vi "PH_O2_Watch.ProcCases.vi"(0 "i ref in":refnum<vi>, 1 "selector":string, 2 "Data":T1, 3 "call cluster":T2={"Object"="", "Selector"="", "CallType"=enum."synchronous", "Async Object"="", "Async Selector"="", "Data Descriptor"="", "Data"=[], "Error #"=0, "Expire"=0}, 5 "error in (no error)":errorcluster) -> (14 "i ref out":refnum<vi>, 17 "answer cluster":T2={"Object"="", "Selector"="", "CallType"=enum."synchronous", "Async Object"="", "Async Selector"="", "Data Descriptor"="", "Data"=[], "Error #"=0, "Expire"=0}, 19 "error out":errorcluster)   [LabVIEW 2014, in "PH_O2_Watch.lvlib"]
doc: "This method is called by a process from within the default case in the event loop. The methods of a class that are linked to events will be called from THIS method. Add your code here."
uses:
  PH_O2_Watch.lvlib
  CSCore/CSSystem/CoreDefs/CoreDefs.call_type.ctl
  CSCore/BaseProcess/BaseProcess.descriptor string definition.ctl
  CSCore/CSSystem/CoreDefs/CoreDefs.rawDataType.ctl
  CSCore/CSSystem/CoreLib/CoreLib.string 2 byte array.vi
  CSCore/CSSystem/CoreLib/CoreLib.byte array 2 double.vi
  CSCore/BaseProcess/BaseProcess.lvlib
  PH_Common/PH_Common.lvlib
  CSCore/CSSystem/CoreLib/CoreLib.lvlib
  CSCore/CAEObj/CAEObj.lvlib
  PH_PSDBWriter/PH_PSDBWriter.lvlib
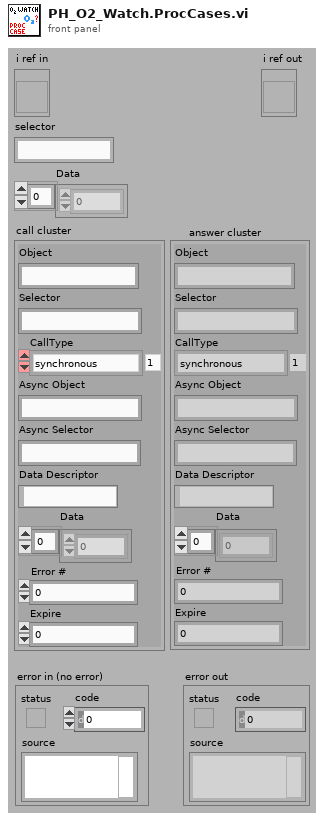
[diagram p1: front panel]
types:
  T1 = typedef "CoreDefs.rawDataType.ctl" = i8[]
  T2 = typedef "CoreDefs.call_type.ctl" = cluster{"Object":string, "Selector":string, "CallType":enum16{"simple", "synchronous", "asynchronous"}, "Async Object":string, "Async Selector":string, "Data Descriptor":T3, "Data":T1, "Error #":i32, "Expire":u32}
  T3 = typedef "BaseProcess.lvlib/BaseProcess.descriptor string definition.ctl" = string
  T4 = typedef "PH_StatusHandler.lvlib/PH_StatusHandler.Status.ctl" = i16
  T5 = typedef "PH_O2_Watch.lvlib/PH_O2_Watch.i attribute.ctl" = cluster{"GUI Refs":cluster{"PreAlert":refnum<vi>, "Alert":refnum<vi>, "Failure":refnum<vi>, "Concentration":refnum<vi>, "Delete":refnum<vi>, "Limit":refnum<vi>}, "State PreAlert":T4, "State Alert":T4, "State Failure":T4, "Concentration":dbl, "Limit":dbl}
  T6 = typedef "PH_PSDBWriter.lvlib/PH_PSDBWriter.PHELIX-Subsystems.ctl" = i32
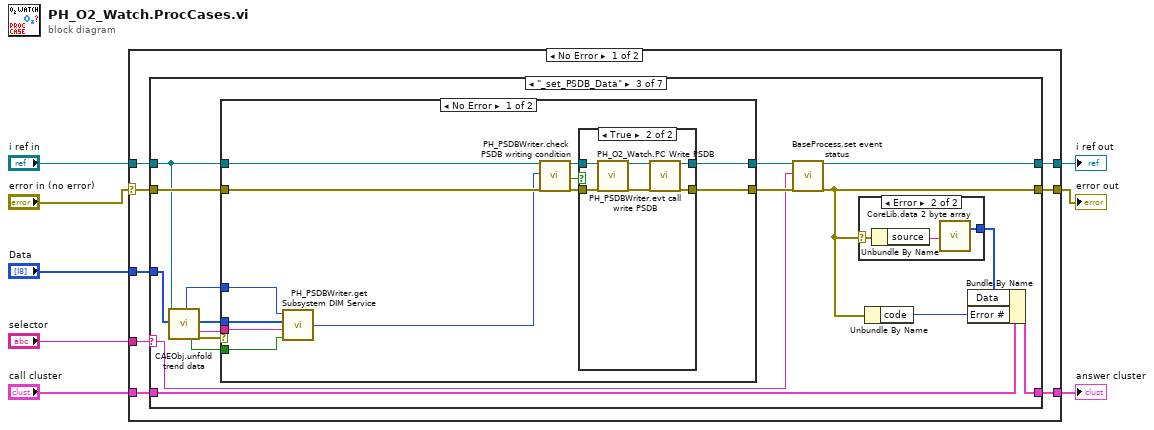
[diagram p0: block diagram]
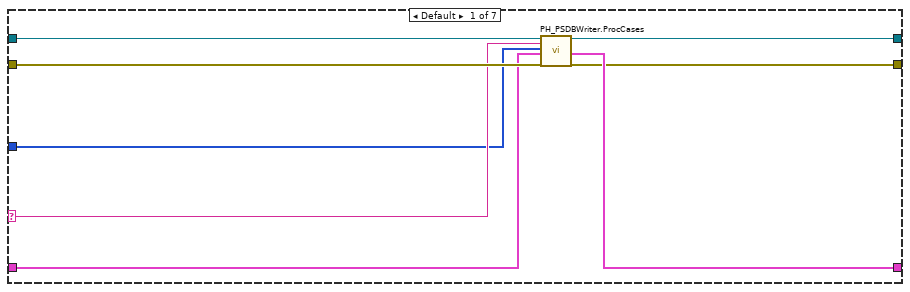
[diagram p2: hidden frame]
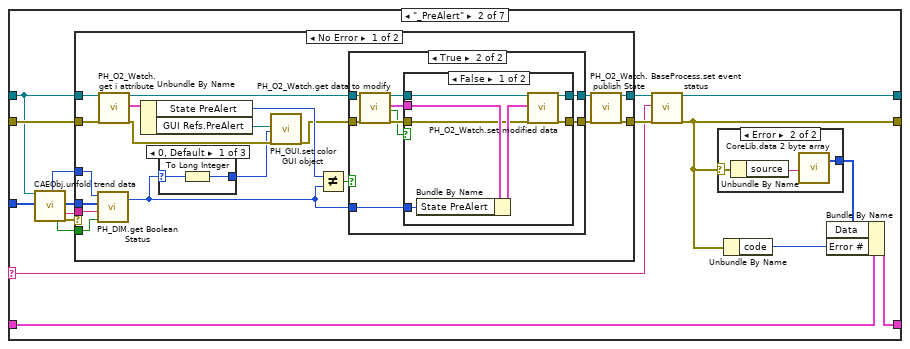
[diagram p3: hidden frame]
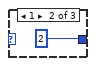
[diagram p5: hidden frame]
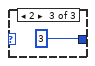
[diagram p6: hidden frame]
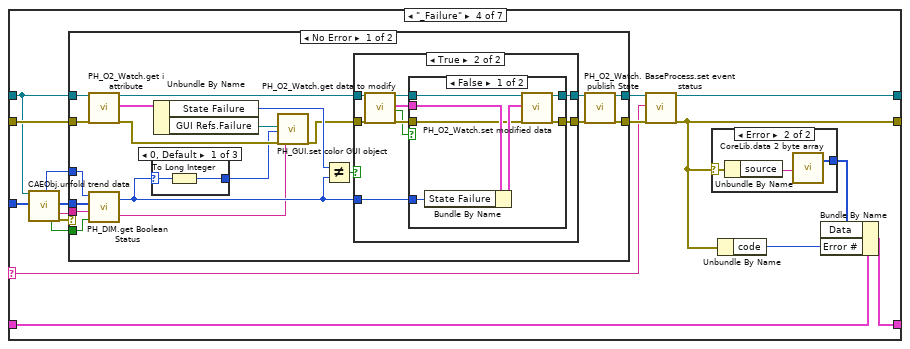
[diagram p13: hidden frame]
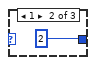
[diagram p15: hidden frame]
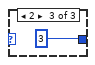
[diagram p16: hidden frame]
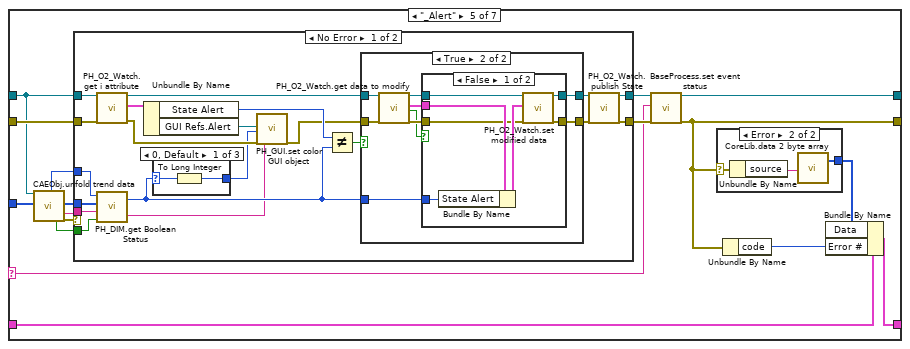
[diagram p20: hidden frame]
diagram:
  n1 = case shown="No Error" "error in (no error)" {
    selector: "error in (no error)" -> [w9 w384]
    tunnel: "selector" -> [w16 _]
    tunnel: [w15 w383] -> w7
    tunnel: "call cluster" -> [w14 w383]
    tunnel: "i ref in" -> [w13 w385]
    tunnel: "Data" -> [w12 _]
    tunnel: [w11 w385] -> w3
    tunnel: [w10 w384] -> w2
    frame No Error {
      n2 = case shown="\"_set_PSDB_Data\"" w16 {
        selector: w16 -> [w21 w30 w90 w138 w203 w268 w332]
        tunnel: w13 -> [w20 w31 w96 w137 w204 w270 w336]
        tunnel: w14 -> [w22 w28 w94 w135 w201 w266 w331]
        tunnel: [w23 w29 w95 w136 w202 w267 w335] -> w15
        tunnel: w9 -> [w24 w32 w97 w139 w205 w271 w337]
        tunnel: w12 -> [w19 w27 w93 w134 w200 w269 _]
        tunnel: [w18 w26 w92 w133 w199 w265 w334] -> w11
        tunnel: [w17 w25 w91 w132 w198 w264 w333] -> w10
        frame Default {
          n3 = call "PH_PSDBWriter.ProcCases.vi"("i ref in"=w20, "selector"=w21, "Data"=w19, "call cluster"=w22, "error in"=w24) -> ("i ref out"=w18:refnum<vi>, "answer cluster"=w23:T2, "error out"=w17:errorcluster)  [unwired: 12 in]
        }
        frame "_PreAlert" {
          n4 = call "CAEObj.unfold trend data.vi"("i ref in"=w31, "raw trend data"=w27) -> ("quality"=w38:i32, "no link"=w37:bool, "data"=w39:i8[], "typeDescriptor"=w40:string, "error out"=w41:errorcluster)  [unwired: 9 in, 4 out]
          n5 = case shown="No Error" w41 {
            tunnel: [w52 w89] -> w34
            tunnel: w31 -> [w58 w89]
            tunnel: w32 -> [w63 w88]
            tunnel: [w50 w88] -> w33
            tunnel: w40 -> [w62 _]
            tunnel: w39 -> [w61 _]
            tunnel: w38 -> [w60 _]
            tunnel: w37 -> [w59 _]
            frame No Error {
              n6 = call "PH_DIM.get Boolean Status.vi"("no link"=w59, "typeDescriptor"=w62, "data"=w61, "quality"=w60) -> ("Status"=w46:T4)  [unwired: 1 out]
              n7 = call "PH_O2_Watch.get i attribute.vi"("i ref in"=w58, "error in (no error)"=w63) -> ("i ref out"=w57:refnum<vi>, "i attribute"=w56:T5, "error out"=w48:errorcluster)  [unwired: 15 in]
              n8 = Unbundle By Name(w56) -> ("State PreAlert"=w55:T4, "GUI Refs.PreAlert"=w49:refnum<vi>)
              n9 = case shown="0, Default" w46 {
                selector: w46 -> [w65 _ _]
                tunnel: [w64 2 3] -> w45
                frame 0, Default {
                  n10 = To Long Integer(number=w65) -> (32bit integer=w64:i32)
                }
                frame 1 {
                }
                frame 2 {
                }
              }
              n11 = call "PH_GUI.set color GUI object.vi"("GUI object Ref"=w49, "State"=w45, "error in (no error)"=w48) -> ("error out"=w47:errorcluster)  [unwired: 16 in]
              n12 = Not Equal?(x=w55, y=w46) -> (x != y?=w54:bool)
              n13 = case shown="True" w54 {
                tunnel: w46 -> [_ w74]
                tunnel: [w69 w71] -> w51
                tunnel: [w68 w70] -> w53
                tunnel: w47 -> [w68 w73]
                tunnel: w57 -> [w69 w72]
                frame False {
                }
                frame True {
                  n14 = call "PH_O2_Watch.get data to modify.vi"("i ref in"=w72, "error in (no error)"=w73) -> ("i ref out"=w77:refnum<vi>, "i attribute"=w78:T5, "timed out"=w75:bool, "error out"=w76:errorcluster)  [unwired: 14 in]
                  n15 = case shown="False" w75 {
                    tunnel: w78 -> [w82 _]
                    tunnel: w74 -> [w80 _]
                    tunnel: [w85 w86] -> w70
                    tunnel: w77 -> [w84 w87]
                    tunnel: [w83 w87] -> w71
                    tunnel: w76 -> [w79 w86]
                    frame False {
                      n16 = Bundle By Name(cluster=w82, "State PreAlert"=w80) -> (w81:T5)
                      n17 = call "PH_O2_Watch.set modified data.vi"("i ref in"=w84, "i attribute"=w81, "error in (no error)"=w79) -> ("i ref out"=w83:refnum<vi>, "error out"=w85:errorcluster)  [unwired: 15 in]
                    }
                    frame True {
                    }
                  }
                }
              }
              n18 = call "PH_O2_Watch.publish State.vi"("i ref in"=w51, "error in (no error)"=w53) -> ("i ref out"=w52:refnum<vi>, "error out"=w50:errorcluster)  [unwired: 16 in]
            }
            frame Error {
            }
          }
          n19 = call "BaseProcess.set event status.vi"("i ref in"=w34, "EventStatus"=w30, "error in (no error)"=w33) -> ("i ref out"=w26:refnum<vi>, "error out"=w25:errorcluster)  [unwired: 14 in, 1 out]
          n20 = case shown="Error" w25 {
            selector: w25 -> [_ w44]
            tunnel: [_ w42] -> w35
            frame No Error {
            }
            frame Error {
              n21 = Unbundle By Name(w44) -> ("source"=w43:string)
              n22 = call-poly "CoreLib.data 2 byte array.vi"("string"=w43) -> ("byteArray out"=w42:T1)  [unwired: 18 in]
            }
          }
          n23 = Unbundle By Name(w25) -> ("code"=w36:i32)
          n24 = Bundle By Name(cluster=w28, "Data"=w35, "Error #"=w36) -> (w29:T2)
        }
        frame "_set_PSDB_Data" {
          n25 = call "CAEObj.unfold trend data.vi"("i ref in"=w96, "raw trend data"=w93) -> ("quality"=w103:i32, "no link"=w102:bool, "data"=w104:i8[], "typeDescriptor"=w105:string, "error out"=w106:errorcluster)  [unwired: 9 in, 4 out]
          n26 = case shown="No Error" w106 {
            tunnel: [w121 w131] -> w99
            tunnel: w96 -> [w117 w131]
            tunnel: w97 -> [w119 w130]
            tunnel: [w120 w130] -> w98
            tunnel: w105 -> [w113 _]
            tunnel: w104 -> [w114 _]
            tunnel: w103 -> [w111 _]
            tunnel: w102 -> [w112 _]
            frame No Error {
              n27 = call "PH_PSDBWriter.get Subsystem DIM Service.vi"("no link"=w112, "typeDescriptor"=w113, "data"=w114, "quality"=w111) -> ("PHELIX Subsystems"=w110:T6)
              n28 = call "PH_PSDBWriter.check PSDB writing condition.vi"("i ref in"=w117, "wanted Subsystem"=w110, "error IO"=w119) -> ("i ref out"=w116:refnum<vi>, "write PSDB?"=w115:bool, "error out"=w118:errorcluster)  [unwired: 14 in]
              n29 = case shown="True" w115 {
                tunnel: [w123 w129] -> w121
                tunnel: [w122 w128] -> w120
                tunnel: w116 -> [w123 w127]
                tunnel: w118 -> [w122 w125]
                frame False {
                }
                frame True {
                  n30 = call "PH_O2_Watch.PC Write PSDB.vi"("i ref in"=w127, "error IO"=w125) -> ("i ref out"=w126:refnum<vi>, "error out"=w124:errorcluster)  [unwired: 16 in]
                  n31 = call "PH_PSDBWriter.evt call write PSDB.vi"("i ref in"=w126, "error in (no error)"=w124) -> ("i ref out"=w129:refnum<vi>, "error out"=w128:errorcluster)  [unwired: 16 in]
                }
              }
            }
            frame Error {
            }
          }
          n32 = call "BaseProcess.set event status.vi"("i ref in"=w99, "EventStatus"=w90, "error in (no error)"=w98) -> ("i ref out"=w92:refnum<vi>, "error out"=w91:errorcluster)  [unwired: 14 in, 1 out]
          n33 = case shown="Error" w91 {
            selector: w91 -> [_ w109]
            tunnel: [_ w107] -> w100
            frame No Error {
            }
            frame Error {
              n34 = Unbundle By Name(w109) -> ("source"=w108:string)
              n35 = call-poly "CoreLib.data 2 byte array.vi"("string"=w108) -> ("byteArray out"=w107:T1)  [unwired: 18 in]
            }
          }
          n36 = Unbundle By Name(w91) -> ("code"=w101:i32)
          n37 = Bundle By Name(cluster=w94, "Data"=w100, "Error #"=w101) -> (w95:T2)
        }
        frame "_Failure" {
          n38 = call "CAEObj.unfold trend data.vi"("i ref in"=w137, "raw trend data"=w134) -> ("quality"=w145:i32, "no link"=w144:bool, "data"=w146:i8[], "typeDescriptor"=w147:string, "error out"=w148:errorcluster)  [unwired: 9 in, 4 out]
          n39 = case shown="No Error" w148 {
            tunnel: [w161 w197] -> w141
            tunnel: w137 -> [w166 w197]
            tunnel: w139 -> [w171 w196]
            tunnel: [w159 w196] -> w140
            tunnel: w147 -> [w170 _]
            tunnel: w146 -> [w169 _]
            tunnel: w145 -> [w168 _]
            tunnel: w144 -> [w167 _]
            frame No Error {
              n40 = call "PH_O2_Watch.get i attribute.vi"("i ref in"=w166, "error in (no error)"=w171) -> ("i ref out"=w165:refnum<vi>, "i attribute"=w164:T5, "error out"=w156:errorcluster)  [unwired: 15 in]
              n41 = call "PH_DIM.get Boolean Status.vi"("no link"=w167, "typeDescriptor"=w170, "data"=w169, "quality"=w168) -> ("further information"=w152:string, "Status"=w154:T4)
              n42 = case shown="0, Default" w154 {
                selector: w154 -> [w173 _ _]
                tunnel: [w172 2 3] -> w153
                frame 0, Default {
                  n43 = To Long Integer(number=w173) -> (32bit integer=w172:i32)
                }
                frame 1 {
                }
                frame 2 {
                }
              }
              n44 = Unbundle By Name(w164) -> ("State Failure"=w163:T4, "GUI Refs.Failure"=w157:refnum<vi>)
              n45 = call "PH_GUI.set color GUI object.vi"("GUI object Ref"=w157, "State"=w153, "error in (no error)"=w156, "Tip Strip (N/A)"=w152) -> ("error out"=w155:errorcluster)  [unwired: 15 in]
              n46 = Not Equal?(x=w163, y=w154) -> (x != y?=w162:bool)
              n47 = case shown="True" w162 {
                tunnel: [w177 w179] -> w160
                tunnel: [w176 w178] -> w158
                tunnel: w155 -> [w176 w182]
                tunnel: w165 -> [w177 w181]
                tunnel: w154 -> [_ w180]
                frame False {
                }
                frame True {
                  n48 = call "PH_O2_Watch.get data to modify.vi"("i ref in"=w181, "error in (no error)"=w182) -> ("i ref out"=w185:refnum<vi>, "i attribute"=w186:T5, "timed out"=w183:bool, "error out"=w184:errorcluster)  [unwired: 14 in]
                  n49 = case shown="False" w183 {
                    tunnel: w186 -> [w190 _]
                    tunnel: w180 -> [w188 _]
                    tunnel: [w193 w194] -> w178
                    tunnel: w185 -> [w192 w195]
                    tunnel: [w191 w195] -> w179
                    tunnel: w184 -> [w187 w194]
                    frame False {
                      n50 = Bundle By Name(cluster=w190, "State Failure"=w188) -> (w189:T5)
                      n51 = call "PH_O2_Watch.set modified data.vi"("i ref in"=w192, "i attribute"=w189, "error in (no error)"=w187) -> ("i ref out"=w191:refnum<vi>, "error out"=w193:errorcluster)  [unwired: 15 in]
                    }
                    frame True {
                    }
                  }
                }
              }
              n52 = call "PH_O2_Watch.publish State.vi"("i ref in"=w160, "error in (no error)"=w158) -> ("i ref out"=w161:refnum<vi>, "error out"=w159:errorcluster)  [unwired: 16 in]
            }
            frame Error {
            }
          }
          n53 = call "BaseProcess.set event status.vi"("i ref in"=w141, "EventStatus"=w138, "error in (no error)"=w140) -> ("i ref out"=w133:refnum<vi>, "error out"=w132:errorcluster)  [unwired: 14 in, 1 out]
          n54 = case shown="Error" w132 {
            selector: w132 -> [_ w151]
            tunnel: [_ w149] -> w142
            frame No Error {
            }
            frame Error {
              n55 = Unbundle By Name(w151) -> ("source"=w150:string)
              n56 = call-poly "CoreLib.data 2 byte array.vi"("string"=w150) -> ("byteArray out"=w149:T1)  [unwired: 18 in]
            }
          }
          n57 = Unbundle By Name(w132) -> ("code"=w143:i32)
          n58 = Bundle By Name(cluster=w135, "Data"=w142, "Error #"=w143) -> (w136:T2)
        }
        frame "_Alert" {
          n59 = call "CAEObj.unfold trend data.vi"("i ref in"=w204, "raw trend data"=w200) -> ("quality"=w211:i32, "no link"=w210:bool, "data"=w212:i8[], "typeDescriptor"=w213:string, "error out"=w214:errorcluster)  [unwired: 9 in, 4 out]
          n60 = case shown="No Error" w214 {
            tunnel: [w224 w263] -> w207
            tunnel: w204 -> [w232 w263]
            tunnel: w205 -> [w237 w262]
            tunnel: [w223 w262] -> w206
            tunnel: w213 -> [w236 _]
            tunnel: w212 -> [w235 _]
            tunnel: w211 -> [w234 _]
            tunnel: w210 -> [w233 _]
            frame No Error {
              n61 = call "PH_O2_Watch.get i attribute.vi"("i ref in"=w232, "error in (no error)"=w237) -> ("i ref out"=w231:refnum<vi>, "i attribute"=w230:T5, "error out"=w222:errorcluster)  [unwired: 15 in]
              n62 = call "PH_DIM.get Boolean Status.vi"("no link"=w233, "typeDescriptor"=w236, "data"=w235, "quality"=w234) -> ("further information"=w218:string, "Status"=w220:T4)
              n63 = Unbundle By Name(w230) -> ("State Alert"=w229:T4, "GUI Refs.Alert"=w227:refnum<vi>)
              n64 = case shown="0, Default" w220 {
                selector: w220 -> [w239 _ _]
                tunnel: [w238 2 4] -> w219
                frame 0, Default {
                  n65 = To Long Integer(number=w239) -> (32bit integer=w238:i32)
                }
                frame 1 {
                }
                frame 2 {
                }
              }
              n66 = call "PH_GUI.set color GUI object.vi"("GUI object Ref"=w227, "State"=w219, "error in (no error)"=w222, "Tip Strip (N/A)"=w218) -> ("error out"=w221:errorcluster)  [unwired: 15 in]
              n67 = Not Equal?(x=w229, y=w220) -> (x != y?=w228:bool)
              n68 = case shown="True" w228 {
                tunnel: w220 -> [_ w248]
                tunnel: [w243 w245] -> w225
                tunnel: [w242 w244] -> w226
                tunnel: w221 -> [w242 w247]
                tunnel: w231 -> [w243 w246]
                frame False {
                }
                frame True {
                  n69 = call "PH_O2_Watch.get data to modify.vi"("i ref in"=w246, "error in (no error)"=w247) -> ("i ref out"=w251:refnum<vi>, "i attribute"=w252:T5, "timed out"=w249:bool, "error out"=w250:errorcluster)  [unwired: 14 in]
                  n70 = case shown="False" w249 {
                    tunnel: w252 -> [w256 _]
                    tunnel: w248 -> [w254 _]
                    tunnel: [w259 w260] -> w244
                    tunnel: w251 -> [w258 w261]
                    tunnel: [w257 w261] -> w245
                    tunnel: w250 -> [w253 w260]
                    frame False {
                      n71 = Bundle By Name(cluster=w256, "State Alert"=w254) -> (w255:T5)
                      n72 = call "PH_O2_Watch.set modified data.vi"("i ref in"=w258, "i attribute"=w255, "error in (no error)"=w253) -> ("i ref out"=w257:refnum<vi>, "error out"=w259:errorcluster)  [unwired: 15 in]
                    }
                    frame True {
                    }
                  }
                }
              }
              n73 = call "PH_O2_Watch.publish State.vi"("i ref in"=w225, "error in (no error)"=w226) -> ("i ref out"=w224:refnum<vi>, "error out"=w223:errorcluster)  [unwired: 16 in]
            }
            frame Error {
            }
          }
          n74 = call "BaseProcess.set event status.vi"("i ref in"=w207, "EventStatus"=w203, "error in (no error)"=w206) -> ("i ref out"=w199:refnum<vi>, "error out"=w198:errorcluster)  [unwired: 14 in, 1 out]
          n75 = case shown="Error" w198 {
            selector: w198 -> [_ w217]
            tunnel: [_ w215] -> w208
            frame No Error {
            }
            frame Error {
              n76 = Unbundle By Name(w217) -> ("source"=w216:string)
              n77 = call-poly "CoreLib.data 2 byte array.vi"("string"=w216) -> ("byteArray out"=w215:T1)  [unwired: 18 in]
            }
          }
          n78 = Unbundle By Name(w198) -> ("code"=w209:i32)
          n79 = Bundle By Name(cluster=w201, "Data"=w208, "Error #"=w209) -> (w202:T2)
        }
        frame "_Concentration" {
          n80 = call "CAEObj.unfold trend data.vi"("i ref in"=w270, "raw trend data"=w269) -> ("quality"=w275:i32, "no link"=w276:bool, "data"=w274:i8[], "typeDescriptor"=w273:string, "error out"=w272:errorcluster)  [unwired: 9 in, 4 out]
          n81 = case shown="No Error" w272 {
            tunnel: [w287 w327] -> w279
            tunnel: [w285 w326] -> w280
            tunnel: w273 -> [w305 _]
            tunnel: w274 -> [w304 _]
            tunnel: w275 -> [w303 _]
            tunnel: w276 -> [w302 _]
            tunnel: w270 -> [w296 w327]
            tunnel: w271 -> [w301 w326]
            frame No Error {
              n82 = call "PH_O2_Watch.get i attribute.vi"("i ref in"=w296, "error in (no error)"=w301) -> ("i ref out"=w295:refnum<vi>, "i attribute"=w294:T5, "error out"=w289:errorcluster)  [unwired: 15 in]
              n83 = call "PH_DIM.get Double.vi"("no link"=w302, "typeDescriptor"=w305, "data"=w304, "quality"=w303) -> ("Value"=w297:dbl)
              n84 = Unbundle By Name(w294) -> ("Concentration"=w293:dbl, "GUI Refs.Concentration"=w291:refnum<vi>)
              n85 = Less?(x=w297, y=0.01) -> (x < y?=w299:bool)
              n86 = Select(t=0.0, s=w299, f=w297) -> (s? t:f=w290:dbl)
              n87 = call "PH_GUI.set double GUI object.vi"("GUI object Ref"=w291, "value"=w290, "error in (no error)"=w289) -> ("error out"=w288:errorcluster)  [unwired: 16 in]
              n88 = Not Equal?(x=w293, y=w290) -> (x != y?=w292:bool)
              n89 = case shown="True" w292 {
                tunnel: w295 -> [w307 w312]
                tunnel: w288 -> [w306 w311]
                tunnel: [w306 w308] -> w284
                tunnel: [w307 w309] -> w286
                tunnel: w290 -> [_ w310]
                frame False {
                }
                frame True {
                  n90 = call "PH_O2_Watch.get data to modify.vi"("i ref in"=w312, "error in (no error)"=w311) -> ("i ref out"=w315:refnum<vi>, "i attribute"=w316:T5, "timed out"=w313:bool, "error out"=w314:errorcluster)  [unwired: 14 in]
                  n91 = case shown="False" w313 {
                    tunnel: w316 -> [w322 _]
                    tunnel: w310 -> [w318 _]
                    tunnel: [w319 w324] -> w308
                    tunnel: w315 -> [w323 w325]
                    tunnel: [w320 w325] -> w309
                    tunnel: w314 -> [w317 w324]
                    frame False {
                      n92 = Bundle By Name(cluster=w322, "Concentration"=w318) -> (w321:T5)
                      n93 = call "PH_O2_Watch.set modified data.vi"("i ref in"=w323, "i attribute"=w321, "error in (no error)"=w317) -> ("i ref out"=w320:refnum<vi>, "error out"=w319:errorcluster)  [unwired: 15 in]
                    }
                    frame True {
                    }
                  }
                }
              }
              n94 = call "PH_O2_Watch.publish State.vi"("i ref in"=w286, "error in (no error)"=w284) -> ("i ref out"=w287:refnum<vi>, "error out"=w285:errorcluster)  [unwired: 16 in]
            }
            frame Error {
            }
          }
          n95 = call "BaseProcess.set event status.vi"("i ref in"=w279, "EventStatus"=w268, "error in (no error)"=w280) -> ("i ref out"=w265:refnum<vi>, "error out"=w264:errorcluster)  [unwired: 14 in, 1 out]
          n96 = case shown="Error" w264 {
            selector: w264 -> [_ w283]
            tunnel: [_ w281] -> w278
            frame No Error {
            }
            frame Error {
              n97 = Unbundle By Name(w283) -> ("source"=w282:string)
              n98 = call-poly "CoreLib.data 2 byte array.vi"("string"=w282) -> ("byteArray out"=w281:T1)  [unwired: 18 in]
            }
          }
          n99 = Unbundle By Name(w264) -> ("code"=w277:i32)
          n100 = Bundle By Name(cluster=w266, "Data"=w278, "Error #"=w277) -> (w267:T2)
        }
        frame "SetLimit" {
          n101 = Unbundle By Name(w331) -> ("Data"=w330:T1)
          n102 = call-poly "CoreLib.byte array 2 data.vi"("byteArray"=w330) -> ("d64"=w328:dbl, "error out"=w329:errorcluster)  [unwired: 16 in, 1 out]
          n103 = case shown="No Error" w329 {
            tunnel: [w348 w382] -> w340
            tunnel: [w345 w380] -> w341
            tunnel: w336 -> [w357 w382]
            tunnel: w337 -> [w358 w381]
            tunnel: w332 -> [_ w379]
            tunnel: w328 -> [w351 _]
            frame No Error {
              n104 = call "PH_O2_Watch.get i attribute.vi"("i ref in"=w357, "error in (no error)"=w358) -> ("i ref out"=w356:refnum<vi>, "i attribute"=w355:T5, "error out"=w350:errorcluster)  [unwired: 15 in]
              n105 = Unbundle By Name(w355) -> ("Limit"=w354:dbl, "GUI Refs.Limit"=w352:refnum<vi>)
              n106 = call "PH_GUI.set double GUI object.vi"("GUI object Ref"=w352, "value"=w351, "error in (no error)"=w350) -> ("error out"=w349:errorcluster)  [unwired: 16 in]
              n107 = Not Equal?(x=w354, y=w351) -> (x != y?=w353:bool)
              n108 = case shown="True" w353 {
                tunnel: [w360 w362] -> w347
                tunnel: [w359 w361] -> w346
                tunnel: w349 -> [w359 w365]
                tunnel: w356 -> [w360 w364]
                tunnel: w351 -> [_ w363]
                frame False {
                }
                frame True {
                  n109 = call "PH_O2_Watch.get data to modify.vi"("i ref in"=w364, "error in (no error)"=w365) -> ("i ref out"=w368:refnum<vi>, "i attribute"=w369:T5, "timed out"=w366:bool, "error out"=w367:errorcluster)  [unwired: 14 in]
                  n110 = case shown="False" w366 {
                    tunnel: w369 -> [w373 _]
                    tunnel: [w376 w377] -> w361
                    tunnel: w368 -> [w375 w378]
                    tunnel: [w374 w378] -> w362
                    tunnel: w367 -> [w370 w377]
                    tunnel: w363 -> [w371 _]
                    frame False {
                      n111 = Bundle By Name(cluster=w373, "Limit"=w371) -> (w372:T5)
                      n112 = call "PH_O2_Watch.set modified data.vi"("i ref in"=w375, "i attribute"=w372, "error in (no error)"=w370) -> ("i ref out"=w374:refnum<vi>, "error out"=w376:errorcluster)  [unwired: 15 in]
                    }
                    frame True {
                    }
                  }
                }
              }
              n113 = call "PH_O2_Watch.publish State.vi"("i ref in"=w347, "error in (no error)"=w346) -> ("i ref out"=w348:refnum<vi>, "error out"=w345:errorcluster)  [unwired: 16 in]
            }
            frame Error {
              n114 = call "CoreLib.set data type mismatch.vi"("error in (no error)"=w381, "error source"=w379) -> ("error out"=w380:errorcluster)  [unwired: 17 in]
            }
          }
          n115 = call "BaseProcess.set event status.vi"("i ref in"=w340, "EventStatus"=w332, "error in (no error)"=w341) -> ("i ref out"=w334:refnum<vi>, "error out"=w333:errorcluster)  [unwired: 14 in, 1 out]
          n116 = case shown="Error" w333 {
            selector: w333 -> [_ w344]
            tunnel: [_ w342] -> w339
            frame No Error {
            }
            frame Error {
              n117 = Unbundle By Name(w344) -> ("source"=w343:string)
              n118 = call-poly "CoreLib.data 2 byte array.vi"("string"=w343) -> ("byteArray out"=w342:T1)  [unwired: 18 in]
            }
          }
          n119 = Unbundle By Name(w333) -> ("code"=w338:i32)
          n120 = Bundle By Name(cluster=w331, "Data"=w339, "Error #"=w338) -> (w335:T2)
        }
      }
    }
    frame Error {
    }
  }
  "answer cluster" <- w7
  "i ref out" <- w3
  "error out" <- w2
